vi "bigcryo_multiRT.vi"() -> ()   [LabVIEW 2019]
panel:
  in  "Folder":path=path "C:/User Data/hlb54/NTS004" caption="Filename"
  in  "File name":string="NTS004"
  out "Action":string="Performing Applied Field Measurement"
  out "B Actual":dbl=0.0985
  out "T Actual":dbl=5.9983
  out "Of":dbl=2.0
  out "Step":dbl
  in  "Reset 2":bool
  in  "Reset":bool
  in  "Keithley":refnum<visa-resource-name>="GPIB1::20::INSTR"
  in  "Lakeshore":refnum<visa-resource-name>="COM7"
  out "R-H 2":cluster{"X":dbl[], "Y":dbl[]}[](graph)=[{"X"=[6.0054, 6.0013, 5.9958, 5.9902, 5.9848, 5.9815, 5.9787, 5.9771, 5.9752, 5.9742, 5.9727, 5.972, 5.9715, 5.9705, 5.9704, 5.9716, 5.9726, 5.9736, 5.9737, 5.9751, 5.9755, 5.9756, 5.9765, 5.9766, 5.9779, 5.9786, 5.9789, 5.9784, 5.9782, 5.9771, 5.9762, 5.9759, 5.9759, 5.9742, 5.9726, 5.9718, 5.9719, 5.9711, 5.9708, 5.9708, 5.9723, 5.9722, 5.973, 5.9732, 5.9734, 5.9734, 5.9723, 5.9716, 5.971, 5.9695, 5.9689, 5.9681, 5.9677, 5.9668, 5.9654, 5.9653, 5.9643, 5.9636, 5.9628, 5.9625, 5.9613, 5.9607, 5.9601], "Y"=[1.81699157, 1.81690907, 1.81660283, 1.81648326, 1.81627202, 1.81593657, 1.81585312, 1.81583345, 1.81562316, 1.81564009, 1.81568468, 1.81557155, 1.81554639, 1.81547141, 1.81553102, 1.81550062, 1.81557465, 1.81561863, 1.81562221, 1.81569743, 1.81575203, 1.81574452, 1.81585658, 1.81596422, 1.81590724, 1.81592166, 1.81598544, 1.81599438, 1.815974, 1.81596053, 1.81583548, 1.81586432, 1.81586516, 1.81574273, 1.81569219, 1.81567919, 1.81552923, 1.8155719, 1.81558704, 1.81555462, 1.81560743, 1.81565726, 1.81563067, 1.81568301, 1.81577587, 1.81566155, 1.81573236, 1.81571484, 1.81553853, 1.81547797, 1.81538594, 1.81534958, 1.81547225, 1.81528556, 1.8154186, 1.81541765, 1.81547093, 1.81536531, 1.81523526, 1.81520331, 1.81510997, 1.81500208, 1.81503594]}] caption="XY Graph"
  out "R-H":cluster{"X":dbl[], "Y":dbl[]}[](graph)=[{"X"=[5.9934, 5.9905, 5.9878, 5.9842, 5.981, 5.9773, 5.976, 5.9759, 5.9758, 5.9754, 5.9753, 5.9746, 5.9749, 5.9742, 5.9733, 5.9728, 5.9718, 5.9702, 5.9695, 5.9691, 5.9683, 5.9679, 5.9679, 5.9672, 5.9661, 5.9649, 5.964, 5.9635, 5.9635, 5.9647, 5.9652, 5.9658, 5.9661, 5.9651, 5.9642, 5.9636, 5.9629, 5.9622, 5.9611, 5.9605], "Y"=[1.81911707, 1.81903112, 1.81899619, 1.819067, 1.81886935, 1.81881952, 1.81872034, 1.81879413, 1.81882036, 1.81876874, 1.81872511, 1.81863272, 1.81870997, 1.81873333, 1.8187089, 1.81863272, 1.81864643, 1.81869745, 1.81878614, 1.8184613, 1.81841743, 1.81854153, 1.81847501, 1.81839752, 1.81870449, 1.81851804, 1.81834447, 1.81827569, 1.81833398, 1.818331, 1.81835544, 1.81836486, 1.81839001, 1.8183285, 1.81825626, 1.81832504, 1.81839526, 1.8183105, 1.81806791, 1.81812811]}] caption="XY Graph"
  in  "Magnet":refnum<visa-resource-name>="COM6"
  in  "dT/dt Warming":dbl=1.0
  in  "GO":bool=TRUE
  in  "dT/dt Cooling":dbl=1.0
  in  "T_min":dbl=5.95
  in  "T_max":dbl=6.0
  in  "Field [T]   Rate [T/min]":dbl[][](array[numeric])=[[0.1, 0.5], [0.15, 0.5]]
  in  "Set Field":bool=TRUE
  in  "App Field":bool=TRUE
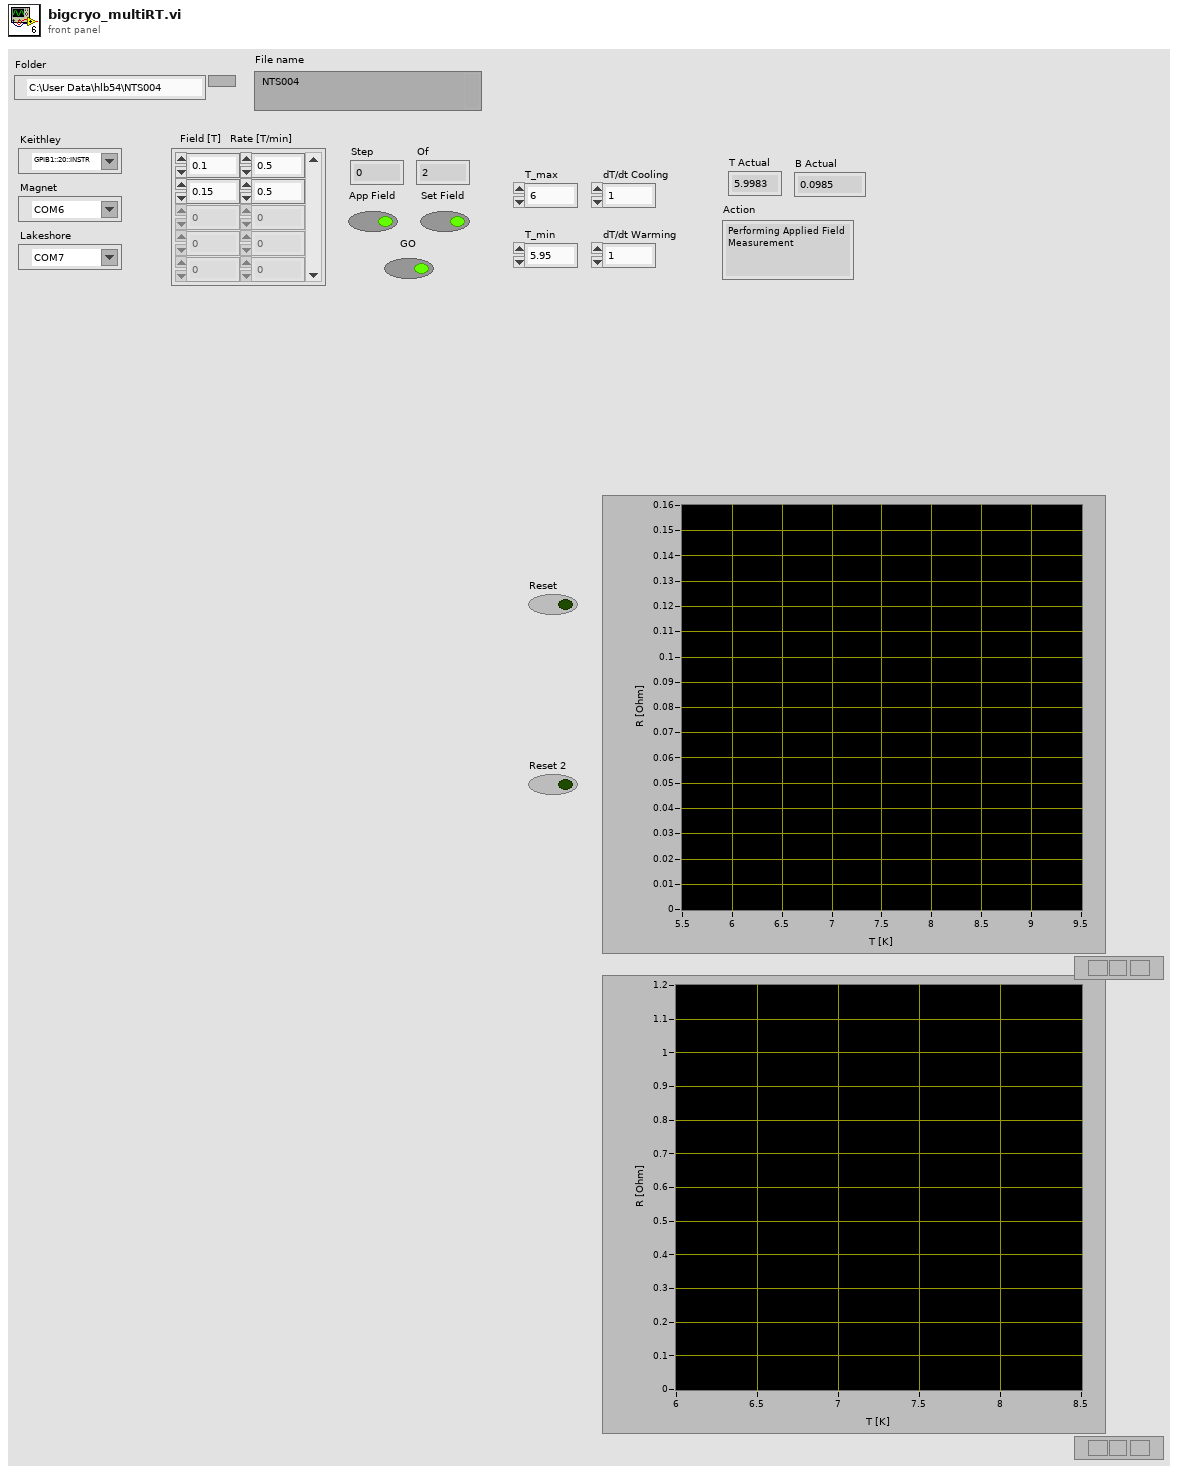
[diagram p1: front panel]
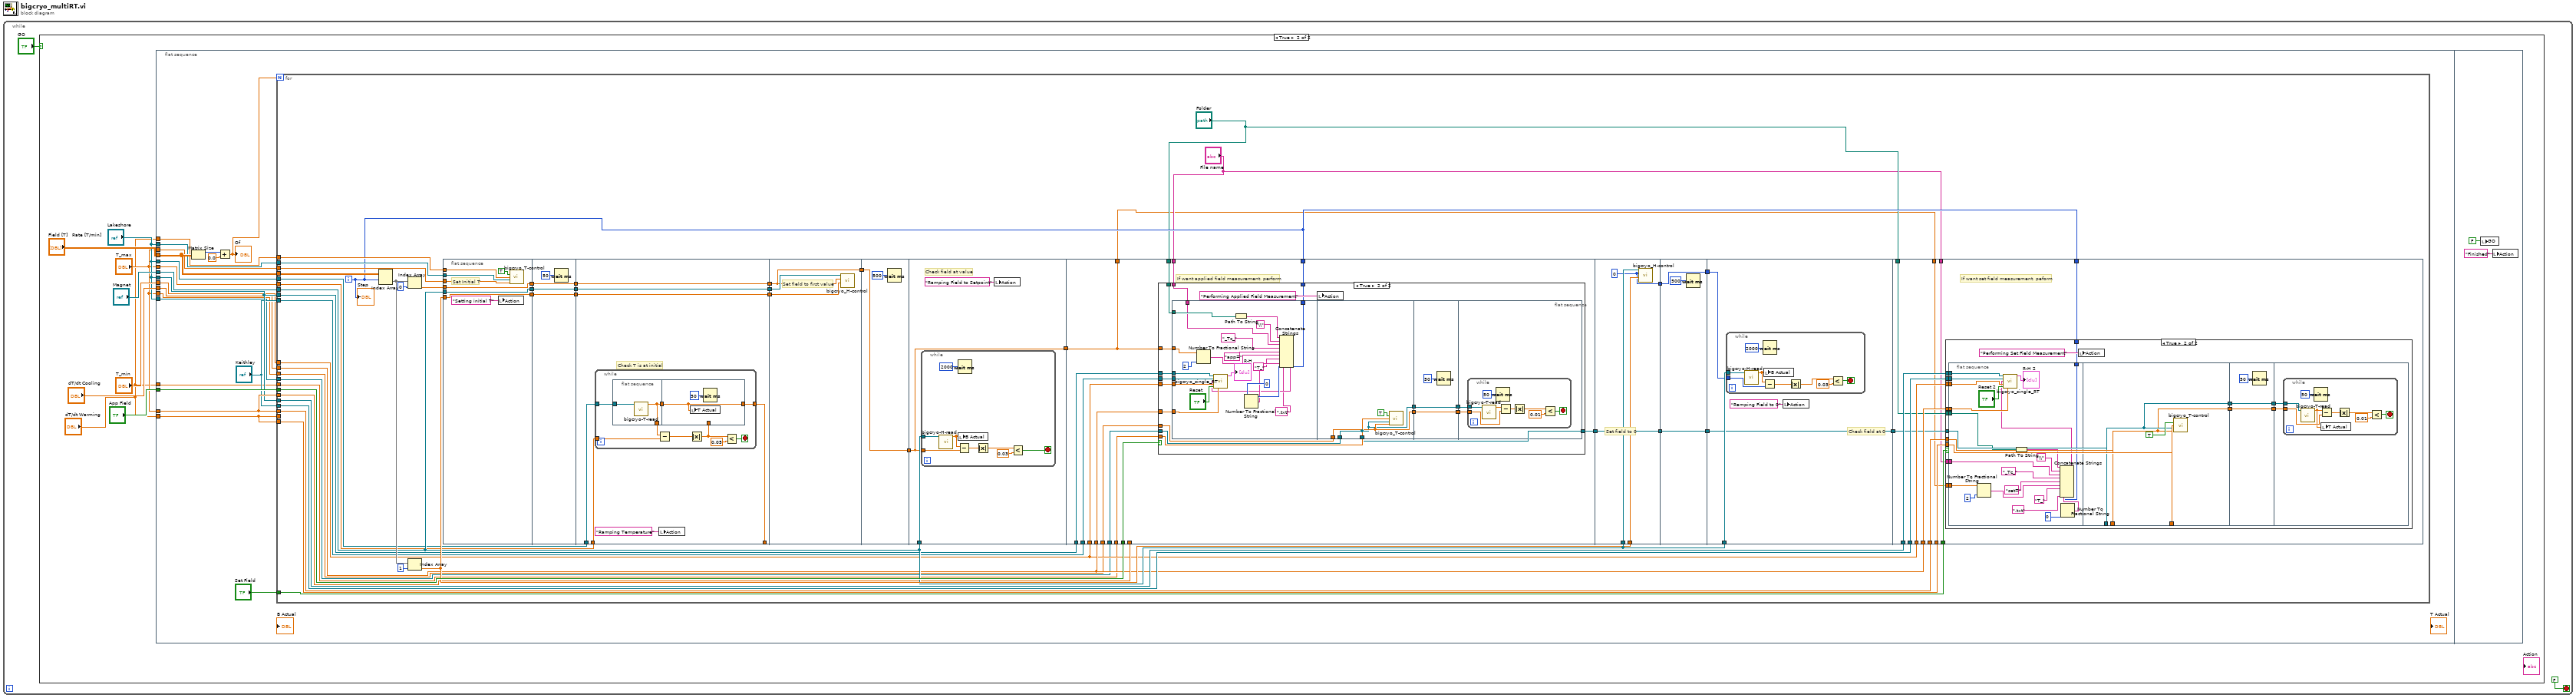
[diagram p0: block diagram]
diagram:
  n1 = while {
    stop <- FALSE stop-if-true
    n2 = case shown="True" "GO" {
      frame False {
      }
      frame True {
        n3 = flat-sequence {
          tunnel: "Field [T]   Rate [T/min]" -> [w22]
          tunnel: "Magnet" -> [w31]
          tunnel: "App Field" -> [w30]
          tunnel: "dT/dt Warming" -> [w28]
          tunnel: "T_max" -> [w27]
          tunnel: "Lakeshore" -> [w26]
          tunnel: "T_min" -> [w24]
          tunnel: "dT/dt Cooling" -> [w23]
          tunnel: "T_max" -> [w20]
          tunnel: "Lakeshore" -> [w19]
          tunnel: "dT/dt Warming" -> [w18]
          tunnel: "Lakeshore" -> [w17]
          tunnel: "T_max" -> [w16]
          tunnel: "Lakeshore" -> [w15]
          tunnel: "T_max" -> [w14]
          tunnel: "dT/dt Warming" -> [w13]
          frame #0 {
            n4 = Matrix Size(0:w22) -> (1:w11:i32)  [unwired: 1 out]
            n5 = Add(x=w11, y=0.0) -> (x+y=w12:dbl)
            "Of" <- w12
            n6 = for {
              N: w12 -> [_]
              tunnel: w22 -> [w76]
              tunnel: w31 -> [w71]
              tunnel: w30 -> [w74]
              tunnel: "Set Field" -> [w73]
              tunnel: w27 -> [w70]
              tunnel: w28 -> [_]
              tunnel: w28 -> [w69]
              tunnel: w27 -> [w68]
              tunnel: w26 -> [w67]
              tunnel: w26 -> [w66]
              tunnel: "Keithley" -> [w65]
              tunnel: "Keithley" -> [w64]
              tunnel: w24 -> [w62]
              tunnel: w23 -> [w63]
              tunnel: w20 -> [w61]
              tunnel: w19 -> [w60]
              tunnel: w18 -> [w59]
              tunnel: w17 -> [w55]
              tunnel: w16 -> [w54]
              tunnel: w15 -> [w53]
              tunnel: w14 -> [w52]
              tunnel: w13 -> [w51]
              i -> [w35]
              n7 = Index Array(array=w76, index (row)=w35) -> (element=w79:dbl[])  [unwired: 1 in]
              n8 = Index Array(array=w79, index=0) -> (element=w75:dbl)
              n9 = Index Array(array=w79, index=1) -> (element=w72:dbl)
              n10 = flat-sequence {
                tunnel: w71 -> [w85]
                tunnel: w75 -> [w86]
                tunnel: w72 -> [w87]
                tunnel: [w87] -> w48
                tunnel: [w86] -> w46
                tunnel: [w85] -> w44
                tunnel: w61 -> [w84]
                tunnel: w60 -> [w83]
                tunnel: w59 -> [w82]
                tunnel: w48 -> [w91]
                tunnel: [w91] -> w47
                tunnel: w46 -> [w90]
                tunnel: [w90] -> w45
                tunnel: w44 -> [w89]
                tunnel: [w89] -> w43
                tunnel: w47 -> [w98]
                tunnel: [w98] -> w58
                tunnel: w45 -> [w97]
                tunnel: [w97] -> w57
                tunnel: w43 -> [w96]
                tunnel: [w96] -> w56
                tunnel: w55 -> [w95]
                tunnel: w54 -> [w94]
                tunnel: [w93] -> _
                tunnel: [w112] -> w42
                tunnel: w58 -> [w114]
                tunnel: w57 -> [w112]
                tunnel: w56 -> [w113]
                tunnel: w42 -> [w116]
                tunnel: [w116] -> w41
                tunnel: w41 -> [w117]
                tunnel: w71 -> [w119]
                tunnel: [w117] -> w36
                tunnel: w74 -> [w140]
                tunnel: w70 -> [_]
                tunnel: w67 -> [w139]
                tunnel: w65 -> [w138]
                tunnel: w62 -> [w137]
                tunnel: w63 -> [w136]
                tunnel: w53 -> [w135]
                tunnel: w52 -> [w134]
                tunnel: w51 -> [w133]
                tunnel: [w132] -> w50
                tunnel: "Folder" -> [w131]
                tunnel: "File name" -> [w130]
                tunnel: w36 -> [w128]
                tunnel: w35 -> [w129]
                tunnel: [w128] -> w32
                tunnel: w72 -> [w199]
                tunnel: w71 -> [w200]
                tunnel: [w198] -> w40
                tunnel: w50 -> [w197]
                tunnel: [w197] -> w38
                tunnel: w40 -> [w203]
                tunnel: [w203] -> w39
                tunnel: w38 -> [w202]
                tunnel: [w202] -> w37
                tunnel: w71 -> [w207]
                tunnel: w39 -> [w206]
                tunnel: w37 -> [w205]
                tunnel: [w205] -> w49
                tunnel: w73 -> [w227]
                tunnel: w69 -> [w226]
                tunnel: w68 -> [w225]
                tunnel: w66 -> [w224]
                tunnel: w64 -> [w223]
                tunnel: w63 -> [w222]
                tunnel: w62 -> [w221]
                tunnel: w49 -> [w220]
                tunnel: w35 -> [w219]
                tunnel: "Folder" -> [w218]
                tunnel: "File name" -> [w217]
                tunnel: w32 -> [w216]
                frame #0 {
                  # "Set Initial T"
                  n11 = local write "Action"("Setting initial T") -> ()
                  n12 = call "bigcryo_T-control.vi"("Ramp Mode"=TRUE, "Rate  [K/min]"=w82, "VISA resource name out"=w83, "Set Sample Temp [K]"=w84) -> ()  [unwired: 12 in]
                }
                frame #1 {
                  n13 = Wait (ms)(milliseconds to wait=50) -> ()  [unwired: 1 out]
                }
                frame #2 {
                  # "Check T is at initial"
                  n14 = while {
                    tunnel: w94 -> [w105]
                    tunnel: w95 -> [w103]
                    tunnel: [w100] -> w93
                    stop <- w104 stop-if-true
                    n15 = flat-sequence {
                      tunnel: w103 -> [w109]
                      tunnel: [w108] -> w102
                      tunnel: [w108] -> w101
                      tunnel: w101 -> [w110]
                      tunnel: [w110] -> w100
                      tunnel: w99 -> [_]
                      frame #0 {
                        n16 = call "bigcryo-T-read.vi"("VISA resource name out"=w109) -> ("Sample Temp [K]"=w108:dbl)  [unwired: 9 in, 1 out]
                      }
                      frame #1 {
                        n17 = local write "T Actual"(w110) -> ()
                        n18 = Wait (ms)(milliseconds to wait=50) -> ()  [unwired: 1 out]
                      }
                    }
                    n19 = Subtract(x=w102, y=w105) -> (x-y=w106:dbl)
                    n20 = Absolute Value(x=w106) -> (abs(x)=w99:dbl)
                    n21 = Less?(x=w99, y=0.05) -> (x < y?=w104:bool)
                  }
                  n22 = local write "Action"("Ramping Temperature") -> ()
                }
                frame #3 {
                  # "Set field to first value"
                  n23 = call "bigcryo_H-control.vi"("Rate [T/min]"=w114, "Set Field [T]"=w112, "Magnet Power supply"=w113) -> ()  [unwired: 9 in]
                }
                frame #4 {
                  n24 = Wait (ms)(milliseconds to wait=500) -> ()  [unwired: 1 out]
                }
                frame #5 {
                  # "Check field at value"
                  n25 = while {
                    tunnel: w117 -> [w124]
                    tunnel: w119 -> [w122]
                    stop <- w123 stop-if-true
                    n26 = call "bigcryo-H-read.vi"("Magnet Power supply"=w122) -> ("Magnetic Field [T]"=w121:dbl)  [unwired: 10 in]
                    n27 = Subtract(x=w121, y=w124) -> (x-y=w125:dbl)
                    n28 = Wait (ms)(milliseconds to wait=2000) -> ()  [unwired: 1 out]
                    n29 = local write "B Actual"(w121) -> ()
                    n30 = Absolute Value(x=w125) -> (abs(x)=w127:dbl)
                    n31 = Less?(x=w127, y=0.03) -> (x < y?=w123:bool)
                  }
                  n32 = local write "Action"("Ramping Field to Setpoint") -> ()
                }
                frame #6 {
                  # "If want applied field measurement, perform"
                  n33 = case shown="True" w140 {
                    tunnel: w139 -> [_ w158]
                    tunnel: w138 -> [_ w157]
                    tunnel: w137 -> [_ w156]
                    tunnel: w136 -> [_ w155]
                    tunnel: w135 -> [w141 w154]
                    tunnel: w134 -> [_ w153]
                    tunnel: w133 -> [_ w152]
                    tunnel: [w141 w151] -> w132
                    tunnel: w131 -> [_ w145]
                    tunnel: w130 -> [_ w144]
                    tunnel: w128 -> [_ w143]
                    tunnel: w129 -> [_ w142]
                    frame False {
                    }
                    frame True {
                      n34 = flat-sequence {
                        tunnel: w158 -> [w178]
                        tunnel: w157 -> [w177]
                        tunnel: w156 -> [w176]
                        tunnel: w155 -> [w175]
                        tunnel: w145 -> [w170]
                        tunnel: w144 -> [w169]
                        tunnel: w143 -> [w167]
                        tunnel: w142 -> [w165]
                        tunnel: w154 -> [w180]
                        tunnel: w153 -> [w181]
                        tunnel: w152 -> [w182]
                        tunnel: [w180] -> w150
                        tunnel: [w181] -> w148
                        tunnel: [w180] -> w151
                        tunnel: w150 -> [w186]
                        tunnel: [w186] -> w149
                        tunnel: w148 -> [w185]
                        tunnel: [w185] -> w147
                        tunnel: w149 -> [w188]
                        tunnel: w147 -> [w187]
                        frame #0 {
                          n35 = Number To Fractional String(number=w167, precision (6)=2) -> (F-format string=w166:string)  [unwired: 2 in]
                          n36 = Path To String(path=w170) -> (string=w173:string)
                          n37 = Number To Fractional String(number=w165, precision (6)=0) -> (F-format string=w163:string)  [unwired: 2 in]
                          n38 = Concatenate Strings(w173, "\\", w169, "_Tc_" ("string"), "app=", w166, "T_" ("string"), w163, ".txt") -> (w161:string)
                          n39 = call "bigcryo_single_RT.vi"("Lake shore"=w178, "Keithley"=w177, "File name"=w161, "Set Sample Temp [K]"=w176, "Reset"="Reset", "Rate  [K/min]"=w175) -> ("R-H"=→"R-H":cluster{"X":dbl[], "Y":dbl[]}[])  [unwired: 7 in, 2 out]
                        }
                        frame #1 {
                          n40 = call "bigcryo_T-control.vi"("Ramp Mode"=TRUE, "Rate  [K/min]"=w182, "VISA resource name out"=w180, "Set Sample Temp [K]"=w181) -> ()  [unwired: 12 in]
                        }
                        frame #2 {
                          n41 = Wait (ms)(milliseconds to wait=50) -> ()  [unwired: 1 out]
                        }
                        frame #3 {
                          n42 = while {
                            tunnel: w187 -> [w193]
                            tunnel: w188 -> [w191]
                            stop <- w192 stop-if-true
                            n43 = call "bigcryo-T-read.vi"("VISA resource name out"=w191) -> ("Sample Temp [K]"=w190:dbl)  [unwired: 9 in, 1 out]
                            n44 = Wait (ms)(milliseconds to wait=50) -> ()  [unwired: 1 out]
                            n45 = Subtract(x=w190, y=w193) -> (x-y=w194:dbl)
                            n46 = Absolute Value(x=w194) -> (abs(x)=w196:dbl)
                            n47 = Less?(x=w196, y=0.01) -> (x < y?=w192:bool)
                          }
                        }
                      }
                      n48 = local write "Action"("Performing Applied Field Measurement") -> ()
                    }
                  }
                }
                frame #7 {
                  w198 = 0
                  # "Set field to 0"
                  n49 = call "bigcryo_H-control.vi"("Rate [T/min]"=w199, "Set Field [T]"=w198, "Magnet Power supply"=w200) -> ()  [unwired: 9 in]
                }
                frame #8 {
                  n50 = Wait (ms)(milliseconds to wait=500) -> ()  [unwired: 1 out]
                }
                frame #9 {
                  # "Check field at 0"
                  n51 = while {
                    tunnel: w207 -> [w211]
                    tunnel: w206 -> [w210]
                    stop <- w212 stop-if-true
                    n52 = call "bigcryo-H-read.vi"("Magnet Power supply"=w211) -> ("Magnetic Field [T]"=w209:dbl)  [unwired: 10 in]
                    n53 = Subtract(x=w209, y=w210) -> (x-y=w213:dbl)
                    n54 = Wait (ms)(milliseconds to wait=2000) -> ()  [unwired: 1 out]
                    n55 = local write "B Actual"(w209) -> ()
                    n56 = Absolute Value(x=w213) -> (abs(x)=w215:dbl)
                    n57 = Less?(x=w215, y=0.03) -> (x < y?=w212:bool)
                  }
                  n58 = local write "Action"("Ramping Field to 0") -> ()
                }
                frame #10 {
                  # "If want set field measurement, peform"
                  n59 = case shown="True" w227 {
                    tunnel: w226 -> [_ w243]
                    tunnel: w225 -> [_ w242]
                    tunnel: w224 -> [_ w241]
                    tunnel: w223 -> [_ w240]
                    tunnel: w222 -> [_ w239]
                    tunnel: w221 -> [_ w238]
                    tunnel: w220 -> [_ w237]
                    tunnel: w219 -> [_ w231]
                    tunnel: w218 -> [_ w230]
                    tunnel: w217 -> [_ w229]
                    tunnel: w216 -> [_ w228]
                    frame False {
                    }
                    frame True {
                      n60 = flat-sequence {
                        tunnel: w241 -> [w263]
                        tunnel: w240 -> [w262]
                        tunnel: w239 -> [w261]
                        tunnel: w238 -> [w260]
                        tunnel: w231 -> [w250]
                        tunnel: w230 -> [w249]
                        tunnel: w229 -> [w248]
                        tunnel: w228 -> [w247]
                        tunnel: w243 -> [w267]
                        tunnel: w242 -> [w265]
                        tunnel: w237 -> [w266]
                        tunnel: [w266] -> w236
                        tunnel: [w265] -> w234
                        tunnel: w236 -> [w271]
                        tunnel: [w271] -> w235
                        tunnel: w234 -> [w270]
                        tunnel: [w270] -> w233
                        tunnel: w235 -> [w273]
                        tunnel: w233 -> [w272]
                        frame #0 {
                          n61 = Number To Fractional String(number=w247, precision (6)=2) -> (F-format string=w254:string)  [unwired: 2 in]
                          n62 = Path To String(path=w249) -> (string=w258:string)
                          n63 = Number To Fractional String(number=w250, precision (6)=0) -> (F-format string=w253:string)  [unwired: 2 in]
                          n64 = Concatenate Strings(w258, "\\", w248, "_Tc_" ("string"), "set=", w254, "T_" ("string"), w253, ".txt") -> (w246:string)
                          n65 = call "bigcryo_single_RT.vi"("Lake shore"=w263, "Keithley"=w262, "File name"=w246, "Set Sample Temp [K]"=w260, "Reset"="Reset 2", "Rate  [K/min]"=w261) -> ("R-H"=→"R-H 2":cluster{"X":dbl[], "Y":dbl[]}[])  [unwired: 7 in, 2 out]
                        }
                        frame #1 {
                          n66 = call "bigcryo_T-control.vi"("Ramp Mode"=TRUE, "Rate  [K/min]"=w267, "VISA resource name out"=w266, "Set Sample Temp [K]"=w265) -> ()  [unwired: 12 in]
                        }
                        frame #2 {
                          n67 = Wait (ms)(milliseconds to wait=50) -> ()  [unwired: 1 out]
                        }
                        frame #3 {
                          n68 = while {
                            tunnel: w272 -> [w278]
                            tunnel: w273 -> [w276]
                            stop <- w277 stop-if-true
                            n69 = call "bigcryo-T-read.vi"("VISA resource name out"=w276) -> ("Sample Temp [K]"=w274:dbl)  [unwired: 9 in, 1 out]
                            n70 = Wait (ms)(milliseconds to wait=50) -> ()  [unwired: 1 out]
                            n71 = Subtract(x=w274, y=w278) -> (x-y=w279:dbl)
                            n72 = local write "T Actual"(w274) -> ()
                            n73 = Absolute Value(x=w279) -> (abs(x)=w281:dbl)
                            n74 = Less?(x=w281, y=0.01) -> (x < y?=w277:bool)
                          }
                        }
                      }
                      n75 = local write "Action"("Performing Set Field Measurement") -> ()
                    }
                  }
                }
              }
              "Step" <- w35
            }
          }
          frame #1 {
            n76 = local write "GO"(FALSE) -> ()
            n77 = local write "Action"("Finished") -> ()
          }
        }
      }
    }
  }
